vi "Get Data.vi"(8 "error in":errorcluster, 11 "eCRDS in":refnum<class "eCRDS.lvclass">) -> (0 "error out":errorcluster, 3 "eCRDS out":refnum<class "eCRDS.lvclass">)   [LabVIEW 2018, in "eCRDS Library.lvlib" / "eCRDS.lvclass"]
doc: "The base CRD <b>Get Data</b> implementation only handles the coadding of traces. If the property <b>Coadd</b> == 1, then this VI will do nothing."
uses:
  eCRDS.lvclass
  C:/Users/Labview/Documents/exscalabar_server/reusable/CRDS/Main/CRDS.lvclass
  C:/Users/Labview/Documents/exscalabar_server/reusable/Instrument/Instrument.lvclass
  eCRDS.lvclass/eCRDS.ctl
  reusable/Instrument/Instrument.lvclass/Instrument.ctl
  reusable/CRDS/Cell/CRDS Cell.lvclass/CRDS Cell.ctl
  reusable/General/Math/Fit Exponential Class/Fit Exponential.lvclass/Fit Exponential.ctl
  <vilib>/DAQmx/read.llb/DAQmx Read (Analog 2D I16 NChan NSamp).vi
  reusable/CRDS/Cell/Write Laser Data.vi
  reusable/CRDS/Cell/Read Data.vi
  reusable/CRDS/Cell/Write Data.vi
  reusable/CRDS/Cell/Read ExpFit.vi
  reusable/General/Math/Fit Exponential Class/Set Dt.vi
  reusable/CRDS/Cell/Write ExpFit.vi
  reusable/Instrument/Read Data.vi
  reusable/Instrument/Write Data.vi
  reusable/CRDS/Data/Cell/CRDS Cell Data.lvclass
  C:/Users/Labview/Documents/exscalabar_server/reusable/Data/Data.lvclass
  <vilib>/DAQmx/miscellaneous.llb/DAQmx Fill In Error Info.vi
  reusable/CRDS/Main/Read Cells.vi
  reusable/Data/Write measTime.vi
  reusable/CRDS/Main/Write Cells.vi
  reusable/CRDS/Cell/CRDS Cell.lvclass
  reusable/Data/Data.lvclass
  reusable/General/Math/Fit Exponential Class/Fit Exponential.lvclass
  reusable/Instrument/Instrument.lvclass
panel:
  out "Array 2":i32[](array[numeric])
  out "Waveform Graph":i16[][](graph)
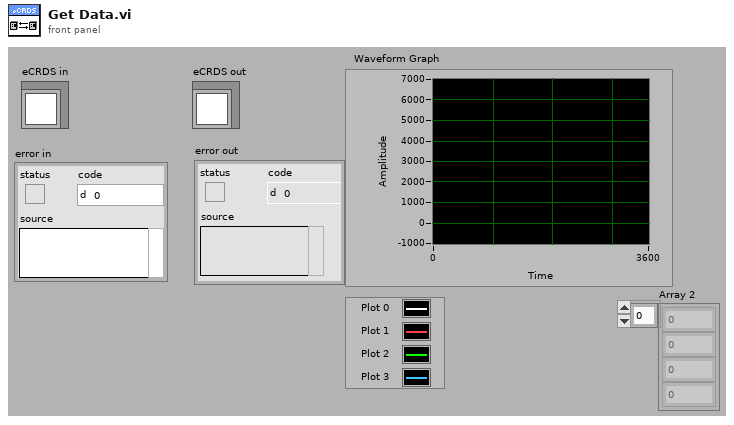
[diagram p1: front panel]
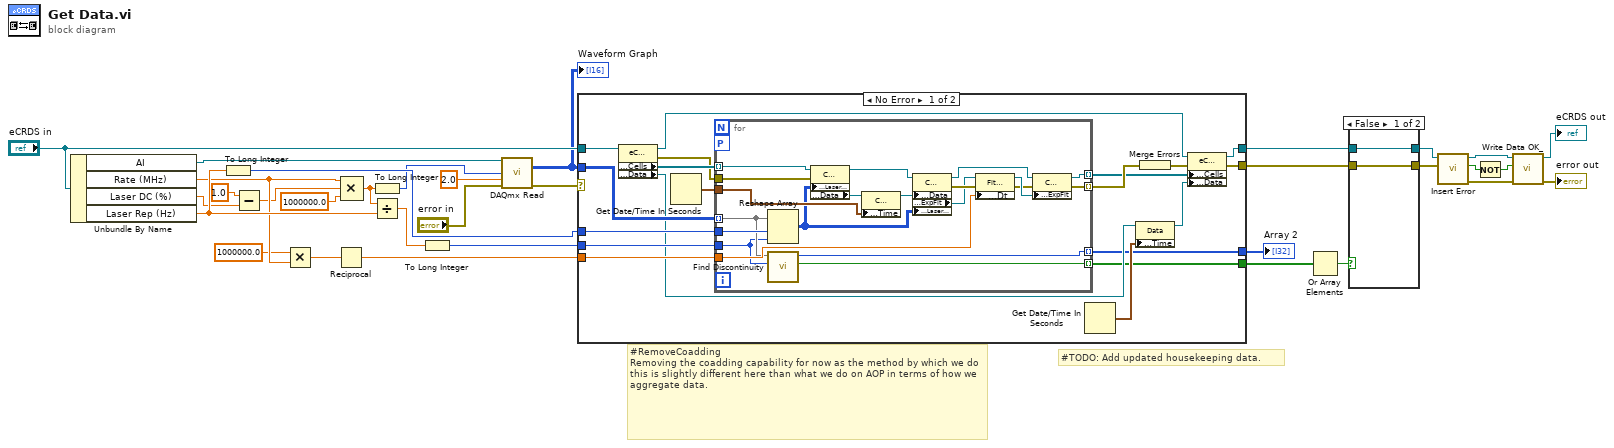
[diagram p0: block diagram]
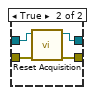
[diagram p2: hidden frame]
diagram:
  # "#TODO: Add updated housekeeping data."
  # "#RemoveCoadding\nRemoving the coadding capability for now as the method by which we do this is slightly different here than what we do on AOP in terms of how we aggregate data."
  n1 = Unbundle By Name("eCRDS in") -> ("AI"=w31:refnum<k21>, "Rate (MHz)"=w16:dbl, "Laser DC (%)"=w8:dbl, "Laser Rep (Hz)"=w27:dbl)
  n2 = To Long Integer(number=w27) -> (32bit integer=w26:i32)
  n3 = Subtract(x=1.0, y=w8) -> (x-y=w9:dbl)
  n4 = Multiply(x=1000000.0 ("y"), y=w16) -> (x*y=w14:dbl)
  n5 = Reciprocal(x=w14) -> (1/x=w17:dbl)
  n6 = Compound Arithmetic op=MULTIPLY(w16, w9, 1000000.0 ("value")) -> (w25:dbl)
  n7 = To Long Integer(number=w25) -> (32bit integer=w13:i32)
  n8 = Divide(x=w25, y=w27) -> (x/y=w29:dbl)
  n9 = To Long Integer(number=w29) -> (32bit integer=w28:i32)
  n10 = call-poly <vilib>:"DAQmx Read.vi"("task/channels in"=w31, "number of samples per channel"=w13, "timeout"=2.0, "error in"="error in") -> ("data"=w7:i16[][], "error out"=w1:errorcluster)  [unwired: 9 in, 1 out]
  "Waveform Graph" <- w7
  n11 = case shown="No Error" w1 {
    selector: w1 -> [_ w73]
    tunnel: [w52 w74] -> w12
    tunnel: w7 -> [w40 _]
    tunnel: "eCRDS in" -> [w51 w74]
    tunnel: w28 -> [w48 _]
    tunnel: w26 -> [w47 _]
    tunnel: [w43 w73] -> w5
    tunnel: w17 -> [w41 _]
    tunnel: [w36 _] -> w11
    tunnel: [w35 _] -> w6
    frame No Error {
      n12 = property class="eCRDS"(reference=w51) -> (reference out=w50:refnum<class "eCRDS.lvclass">, error out=w46:errorcluster, "Data Access:Cells"=w49:refnum<class "CRDS Cell.lvclass">[], "Accessors:Data"=w39:refnum<class "Data.lvclass">)  [unwired: 1 in]
      n13 = Get Date/Time In Seconds() -> (seconds since 1Jan1904=w42:timestamp)
      n14 = for {
        tunnel: w40 -> [w57] mode=indexing
        tunnel: w48 -> [w56]
        tunnel: w47 -> [w72]
        tunnel: w49 -> [w71] mode=indexing
        tunnel: [w59] -> w34 mode=indexing
        workers-P: _ -> [_]
        tunnel: w46 -> [w70]
        tunnel: [w58] -> w45 mode=indexing
        tunnel: w42 -> [w66]
        tunnel: w41 -> [w60]
        tunnel: [w55] -> w36 mode=indexing
        tunnel: [w53] -> w35 mode=indexing
        n15 = Reshape Array(w57, w72, w56) -> (w54:i16[][])
        n16 = call "Find Discontinuity.vi"("Single Record"=w56, "Data"=w57) -> ("Discontinuity Detected"=w55:bool, "cIndex"=w53:i32)  [unwired: 8 in]
        n17 = property class="CRDS Cell"(reference=w71, error in=w70, "Accessors:Laser Data"=w54) -> (reference out=w69:refnum<class "CRDS Cell.lvclass">, "Accessors:Data"=w68:refnum<class "CRDS Cell Data.lvclass">)  [unwired: 1 out]
        n18 = property class="CRDS Cell"(reference=w68, "Accessors:Time"=w66) -> (reference out=w67:refnum<class "CRDS Cell Data.lvclass">)  [unwired: 1 in, 1 out]
        n19 = property class="CRDS Cell"(reference=w69, "Accessors:Data"=w67, "Accessors:Laser Data"=w54) -> (reference out=w63:refnum<class "CRDS Cell.lvclass">, error out=w62:errorcluster, "Accessors:ExpFit"=w61:refnum<class "Fit Exponential.lvclass">)  [unwired: 1 in]
        n20 = property class="Fit Exp"(reference=w61, error in=w62, "Accessors:Dt"=w60) -> (reference out=w65:refnum<class "Fit Exponential.lvclass">, error out=w64:errorcluster)
        n21 = property class="CRDS Cell"(reference=w63, error in=w64, "Accessors:ExpFit"=w65) -> (reference out=w59:refnum<class "CRDS Cell.lvclass">, error out=w58:errorcluster)
      }
      n22 = Get Date/Time In Seconds() -> (seconds since 1Jan1904=w37:timestamp)
      n23 = property class="Data"(reference=w39, "Accessors:Time"=w37) -> (reference out=w38:refnum<class "Data.lvclass">)  [unwired: 1 in, 1 out]
      n24 = Merge Errors(w45) -> (w44:errorcluster)
      n25 = property class="eCRDS"(reference=w50, error in=w44, "Data Access:Cells"=w34, "Accessors:Data"=w38) -> (reference out=w52:refnum<class "eCRDS.lvclass">, error out=w43:errorcluster)
    }
    frame Error {
    }
  }
  "Array 2" <- w6
  n26 = Or Array Elements(Boolean array=w11) -> (logical OR=w2:bool)
  n27 = case shown="False" w2 {
    tunnel: w12 -> [w76 w80]
    tunnel: w5 -> [w75 w79]
    tunnel: [w75 w78] -> w4
    tunnel: [w76 w77] -> w3
    frame False {
    }
    frame True {
      n28 = call "Reset Acquisition.vi"("error in"=w79, "eCRDS in"=w80) -> ("error out"=w78:errorcluster, "eCRDS out"=w77:refnum<class "eCRDS.lvclass">)  [unwired: 8 in]
    }
  }
  n29 = call "Insert Error.vi"("err"=w4, "Instrument in"=w3) -> ("error out"=w21:errorcluster, "error?"=w22:bool, "Instrument out"=w23:refnum<class "eCRDS.lvclass">)  [unwired: 7 in]
  n30 = Not(x=w22) -> (.not. x?=w18:bool)
  n31 = call "Write Data OK_.vi"("error in (no error)"=w21, "Data OK?"=w18, "Instrument in"=w23) -> ("error out"=→"error out":errorcluster, "Instrument out"=→"eCRDS out":refnum<class "eCRDS.lvclass">)  [unwired: 7 in]
